vi "get_status_max-min_wavelength.vi"(8 "error in (no error)":errorcluster, 11 "LightSourceMH110124MaiTai in":refnum<class "LightSourceMH110124MaiTai.lvclass">) -> (0 "error out":errorcluster, 1 "maximal wavelength out":dbl[unit], 2 "minimal wavelength out":dbl[unit], 3 "LightSourceMH110124MaiTai out":refnum<class "LightSourceMH110124MaiTai.lvclass">)   [LabVIEW 2010, in "LightSourceMH110124MaiTai.lvclass"]
uses:
  LightSourceMH110124MaiTai.lvclass
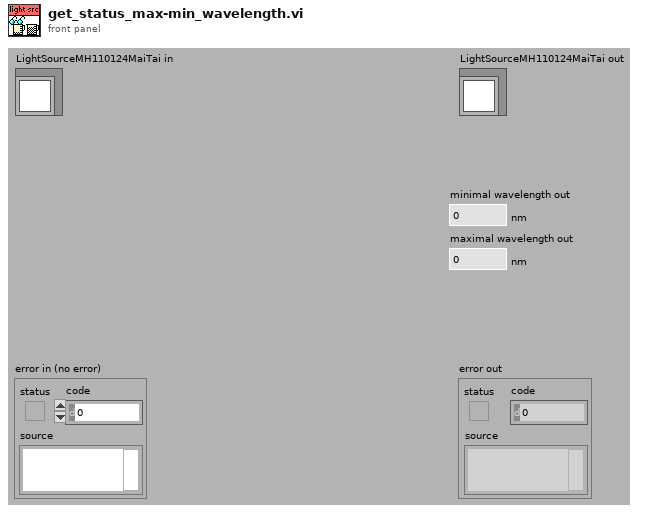
[diagram p1: front panel]
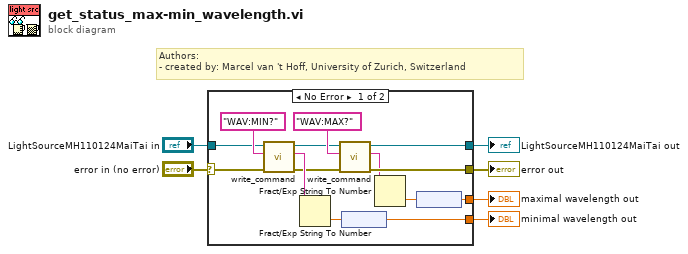
[diagram p0: block diagram]
diagram:
  # "Authors: \n- created by: Marcel van 't Hoff, University of Zurich, Switzerland"
  n1 = case shown="No Error" "error in (no error)" {
    selector: "error in (no error)" -> [w8 w22]
    tunnel: [w19 w22] -> w3
    tunnel: [w20 w21] -> w4
    tunnel: "LightSourceMH110124MaiTai in" -> [w11 w21]
    tunnel: [w15 _] -> w2
    tunnel: [w7 _] -> w1
    frame No Error {
      n2 = call-dynamic "write_command.vi"("error in (no error)"=w8, "string to write"="WAV:MIN?", "LightSourceMH110124MaiTai in"=w11) -> ("error out"=w9:errorcluster, "read string"=w14:string, "LightSourceMH110124MaiTai out"=w10:refnum<class "LightSourceMH110124MaiTai.lvclass">)  [unwired: 6 in]
      n3 = Fract/Exp String To Number(string=w14) -> (number=w13:dbl)  [unwired: 3 in, 1 out]
      n4 = call-dynamic "write_command.vi"("error in (no error)"=w9, "string to write"="WAV:MAX?", "LightSourceMH110124MaiTai in"=w10) -> ("error out"=w19:errorcluster, "read string"=w16:string, "LightSourceMH110124MaiTai out"=w20:refnum<class "LightSourceMH110124MaiTai.lvclass">)  [unwired: 6 in]
      n5 = node(w13) -> (w7:dbl[unit])
      n6 = Fract/Exp String To Number(string=w16) -> (number=w17:dbl)  [unwired: 3 in, 1 out]
      n7 = node(w17) -> (w15:dbl[unit])
    }
    frame Error {
    }
  }
  "error out" <- w3
  "LightSourceMH110124MaiTai out" <- w4
  "maximal wavelength out" <- w2
  "minimal wavelength out" <- w1
